vi "zmq msg data.vi"(8 "error in (no error)":errorcluster, 11 "msg_":T1) -> (0 "error out":errorcluster, 2 "function return":u32, 3 "msg_ out":T1)   [LabVIEW 2025, in "LibZMQ.lvlib"]
doc: "ZMQ_EXPORT void *zmq_msg_data (zmq_msg_t *msg_);"
uses:
  LibZMQ.lvlib
  LV/LibZMQ/libzmq/lv_x86/bin/Release/libzmq-v143-mt-4_3_6.dll
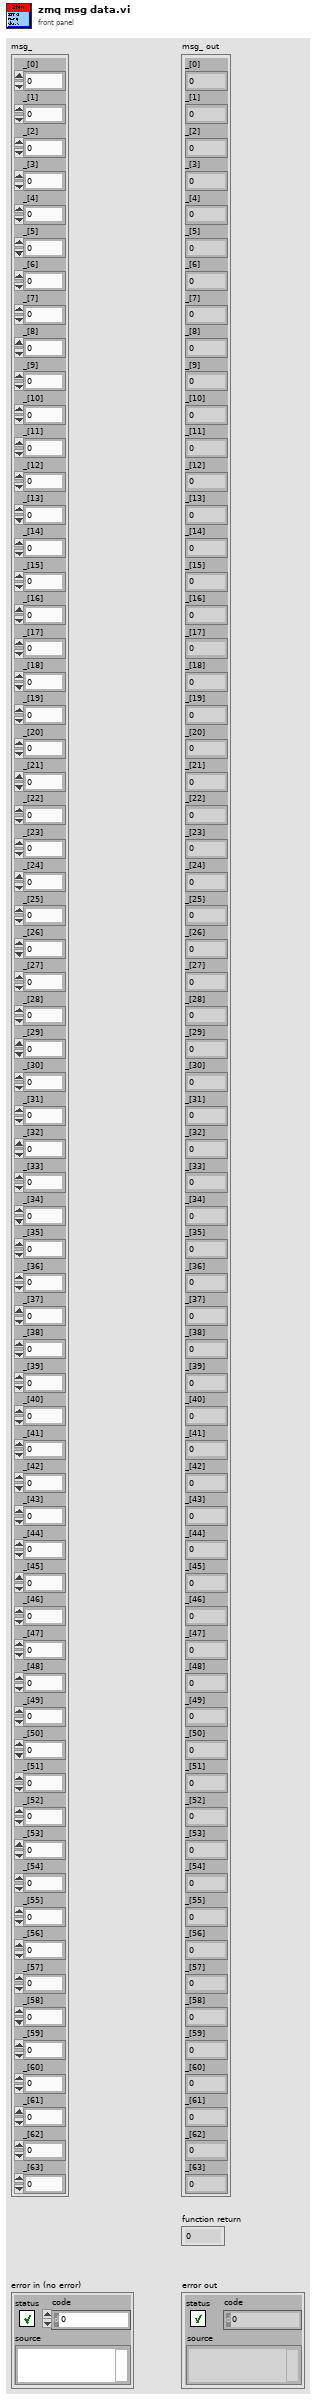
[diagram p1: front panel]
types:
  T1 = cluster{"_[0]":u8, "_[1]":u8, "_[2]":u8, "_[3]":u8, "_[4]":u8, "_[5]":u8, "_[6]":u8, "_[7]":u8, "_[8]":u8, "_[9]":u8, "_[10]":u8, "_[11]":u8, "_[12]":u8, "_[13]":u8, "_[14]":u8, "_[15]":u8, "_[16]":u8, "_[17]":u8, "_[18]":u8, "_[19]":u8, "_[20]":u8, "_[21]":u8, "_[22]":u8, "_[23]":u8, "_[24]":u8, "_[25]":u8, "_[26]":u8, "_[27]":u8, "_[28]":u8, "_[29]":u8, "_[30]":u8, "_[31]":u8, "_[32]":u8, "_[33]":u8, "_[34]":u8, "_[35]":u8, "_[36]":u8, "_[37]":u8, "_[38]":u8, "_[39]":u8, "_[40]":u8, "_[41]":u8, "_[42]":u8, "_[43]":u8, "_[44]":u8, "_[45]":u8, "_[46]":u8, "_[47]":u8, "_[48]":u8, "_[49]":u8, "_[50]":u8, "_[51]":u8, "_[52]":u8, "_[53]":u8, "_[54]":u8, "_[55]":u8, "_[56]":u8, "_[57]":u8, "_[58]":u8, "_[59]":u8, "_[60]":u8, "_[61]":u8, "_[62]":u8, "_[63]":u8}
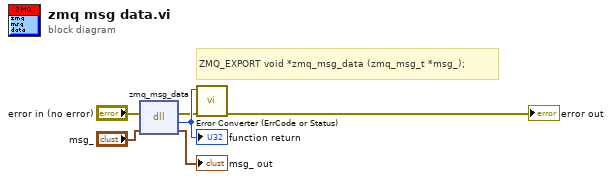
[diagram p0: block diagram]
diagram:
  # "ZMQ_EXPORT void *zmq_msg_data (zmq_msg_t *msg_);"
  n1 = dll-call lib="C:/LV/LibZMQ/libzmq/lv_x86/bin/Release/libzmq-v143-mt-4_3_6.*" fn="zmq_msg_data"(error in="error in (no error)", "msg_"="msg_") -> (error out=w2:errorcluster, w6:u32, "msg_"=→"msg_ out":T1)  [unwired: 2 in, 1 out]
  "function return" <- w6
  n2 = call "Error Converter (ErrCode or Status).vi"("error in (no error)"=w2, "error code"=w6) -> ("error out"=→"error out":errorcluster)  [unwired: 9 in]
